vi "findbuoyVA.vi"(7 "error in":errorcluster) -> (20 "Circles Data (Circle Detection 1)":T2(array[cluster]), 27 "error out":errorcluster)   [LabVIEW 2014]
uses:
  <vilib>/vision/NI_Vision_Development_Module.lvlib
panel:
  in  "File Path":path=path "C:/Users/reggert/Box Sync/Olin/Year III/Robotics/RoboticsVC/Project 4 -- THINK Lab/Think Lab Labview Code Rev B/pool image wall and buoy.png"
  out "Image Out":T1(plugin-control)
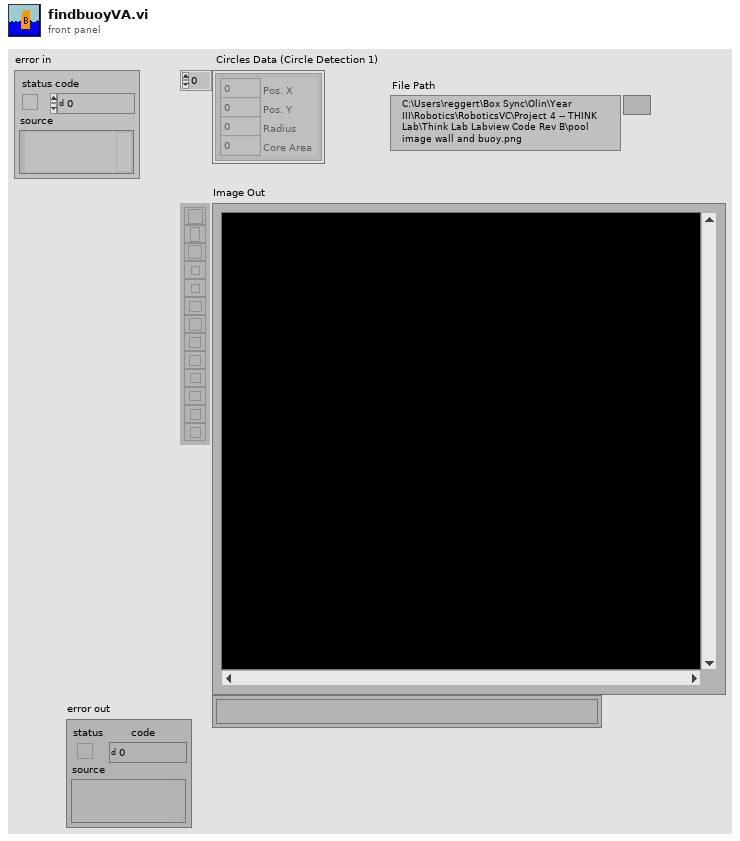
[diagram p1: front panel]
types:
  T1 = typedef "IMAQ Image.ctl" = refnum<image>
  T2 = cluster{"Pos. X":i32, "Pos. Y":i32, "Radius":i32, "Core Area":i32}[]
  T3 = typedef "Image Type" = u32
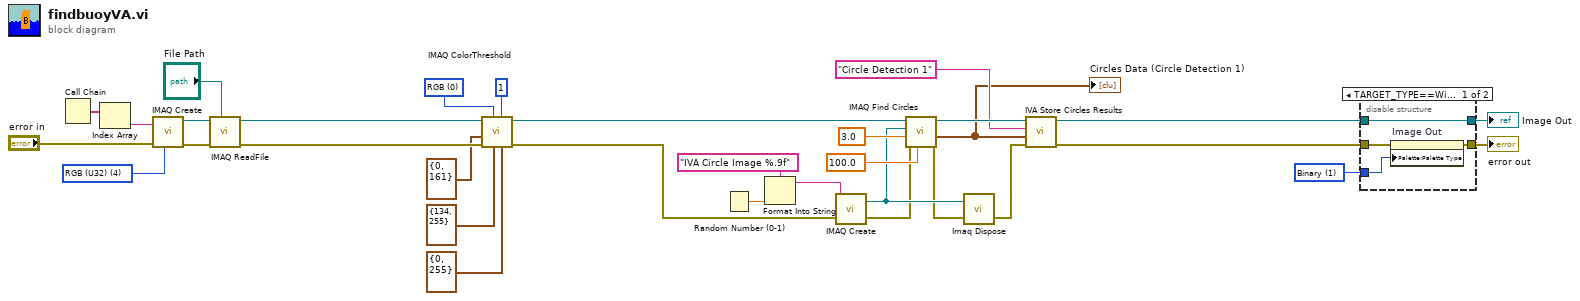
[diagram p0: block diagram]
diagram:
  w2 = u32 1 items=["Grayscale", "Binary", "Gradient", "Rainbow", "Temperature", "User Defined"] ("Palette")
  w24 = u16 0 items=["RGB", "HSL", "HSV", "HSI"] ("Color Mode")
  w26 = T3 4 items=["Grayscale (U8)", "Grayscale (I16)", "Grayscale (SGL)", "Complex (CSG)", "RGB (U32)", "HSL (U32)", "RGB (U64)", "Grayscale (U16)"] ("Image Type")
  n1 = Call Chain() -> (call chain=w28:string[])
  n2 = Index Array(array=w28) -> (element=w27:string)  [unwired: 1 in]
  n3 = call "IMAQ Create"("Image Name"=w27, "Image Type"=w26, "error in (no error)"="error in") -> ("New Image"=w31:T1, "error out"=w30:errorcluster)  [unwired: 1 in, 1 out]
  n4 = call "IMAQ ReadFile"("File Path"="File Path", "error in (no error)"=w30, "Image"=w31) -> ("error out"=w32:errorcluster, "Image Out"=w20:T1)  [unwired: 2 in, 5 out]
  n5 = call "IMAQ ColorThreshold"("Blue or Luma or Val or Inten Range"=cluster{"Lower value":i32, "Upper value":i32} {"Lower value"=0, "Upper value"=255}, "Replace Value"=1, "Green or Sat Range"=cluster{"Lower value":i32, "Upper value":i32} {"Lower value"=134, "Upper value"=255}, "Color Mode"=w24, "error in (no error)"=w32, "Red or Hue Range"=cluster{"Lower value":i32, "Upper value":i32} {"Lower value"=0, "Upper value"=161}, "Image Src"=w20) -> ("error out"=w19:errorcluster, "Image Dst Out"=w11:T1)  [unwired: 1 in, 2 out]
  n6 = Random Number (0-1)() -> (number: 0 to 1=w6:dbl)
  n7 = Format Into String(format string="IVA Circle Image %.9f" ("Image Name"), w6) -> (resulting string=w8:string)  [unwired: 2 in, 1 out]
  n8 = call "IMAQ Create"("Image Name"=w8, "error in (no error)"=w19) -> ("New Image"=w16:T1, "error out"=w15:errorcluster)  [unwired: 2 in, 1 out]
  n9 = call "IMAQ Find Circles"("Max Radius"=sgl 100.0, "error in (no error)"=w15, "Min Radius"=sgl 3.0, "Image Dst"=w16, "Image Src"=w11) -> ("error out"=w14:errorcluster, "Circles Data"=w9:T2)  [unwired: 5 out]
  "Circles Data (Circle Detection 1)" <- w9
  n10 = call "Imaq Dispose"("Image"=w16, "error in (no error)"=w14) -> ("error out"=w13:errorcluster)  [unwired: 1 in, 3 out]
  n11 = call <vilib>:"IVA Store Circles Results.vi"("error in (no error)"=w13, "Circles Data"=w9, "Step Name"="Circle Detection 1", "Image in"=w11) -> ("error out"=w12:errorcluster, "Image dup"=w4:T1)  [unwired: 6 out]
  n12 = disable-structure "Conditional Disable Structure" shown="TARGET_TYPE==Windows" {
    disable-tunnel: w12 -> [w36 w37]
    disable-tunnel: [w35 w37] -> w5
    disable-tunnel: w4 -> [w34 w38]
    disable-tunnel: [w34 w38] -> w3
    disable-tunnel: w2 -> [w33 _]
    frame condition #0 (active) {
      n13 = property on="Image Out" class="ImageControl"(error in=w36, "Palette:Palette Type"=w33) -> (error out=w35:errorcluster)  [unwired: 1 in, 1 out]
    }
    frame condition #1 {
    }
  }
  "error out" <- w5
  "Image Out" <- w3
